vi "Post Exec Callout.vi"(8 "error in (no error)":errorcluster, 11 "Voltage with Step in":refnum<class "Voltage with Step.lvclass">) -> (0 "error out":errorcluster, 3 "Voltage with Step out":refnum<class "Voltage with Step.lvclass">)   [LabVIEW 2023, in "HAF.lvlib" / "Voltage with Step.lvclass"]
doc: "Called at the end of the Processing of a specific Command so that additional code can be run. Adds the step to the current Voltage level and saves it back to the Command."
uses:
  Voltage with Step.lvclass
  Voltage with Step.lvclass/Voltage with Step.ctl
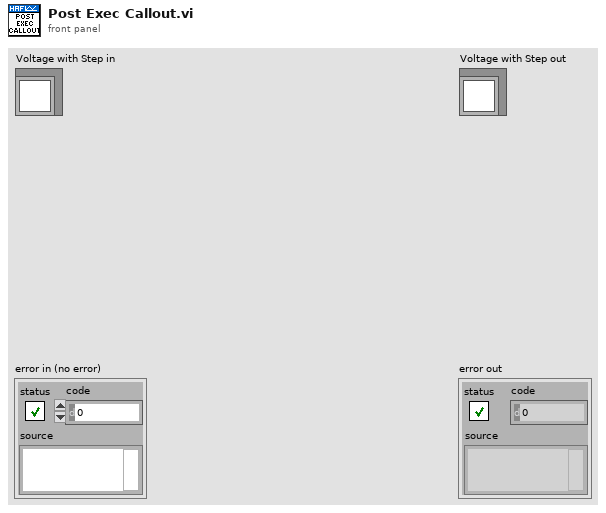
[diagram p1: front panel]
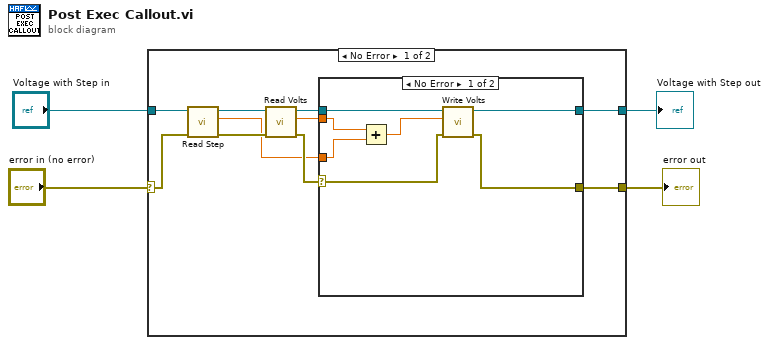
[diagram p0: block diagram]
diagram:
  n1 = case shown="No Error" "error in (no error)" {
    selector: "error in (no error)" -> [w13 w24]
    tunnel: "Voltage with Step in" -> [w14 w25]
    tunnel: [w7 w25] -> w2
    tunnel: [w6 w24] -> w1
    frame No Error {
      n2 = call-dynamic "Read Step.vi"("error in (no error)"=w13, "Voltage with Increment in"=w14) -> ("error out"=w11:errorcluster, "Step"=w5:dbl, "Voltage with Increment out"=w12:refnum<class "Voltage with Step.lvclass">)  [unwired: 7 in]
      n3 = call-dynamic "Read Volts.vi"("error in (no error)"=w11, "Voltage in"=w12) -> ("error out"=w8:errorcluster, "Volts"=w9:dbl, "Voltage out"=w10:refnum<class "Voltage with Step.lvclass">)  [unwired: 7 in]
      n4 = case shown="No Error" w8 {
        selector: w8 -> [w17 w22]
        tunnel: w10 -> [w19 w23]
        tunnel: w9 -> [w21 _]
        tunnel: [w16 w23] -> w7
        tunnel: [w15 w22] -> w6
        tunnel: w5 -> [w20 _]
        frame No Error {
          n5 = Add(x=w21, y=w20) -> (x+y=w18:dbl)
          n6 = call-dynamic "Write Volts.vi"("error in (no error)"=w17, "Volts"=w18, "Voltage in"=w19) -> ("error out"=w15:errorcluster, "Voltage out"=w16:refnum<class "Voltage with Step.lvclass">)  [unwired: 7 in]
        }
        frame Error {
        }
      }
    }
    frame Error {
    }
  }
  "error out" <- w1
  "Voltage with Step out" <- w2
